vi "CVT I32 IndexRead.vi"(3 "error in (no error)":errorcluster, 5 "Tag Index":i32) -> (0 "error out":errorcluster, 1 "Value":i32)   [LabVIEW 2020, in "Current Value Table(Rebuild).lvlib"]
uses:
  Current Value Table(Rebuild).lvlib
  DataTypes/I32_Read Index.vi
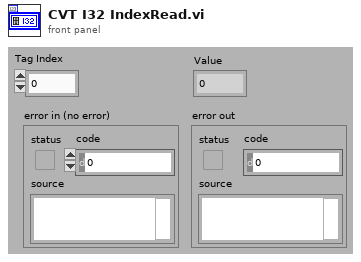
[diagram p1: front panel]
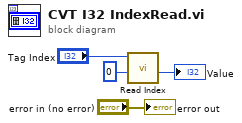
[diagram p0: block diagram]
diagram:
  n1 = call-poly "Read Index.vi"("Default"=0, "Index"="Tag Index") -> ("Value"=→"Value":i32)  [unwired: 9 in]
  "error out" <- "error in (no error)"
